vi "DiffDriveBegin.vi"(8 "error in (no error)":errorcluster) -> (0 "error out":errorcluster)   [LabVIEW 2025]
uses:
  <vilib>/Rock Robotics/WPI/ThirdParty/Phoenix-LabVIEW/Motor Controller/Controls/CTRE_Phoenix_MotorControl_NeutralMode.ctl
  <vilib>/Rock Robotics/WPI/ThirdParty/Phoenix-LabVIEW/Motor Controller/Get/CTRE_Phoenix_MotorController_GetGeneralStatus.vi
  DiffDriveGlobals.vi
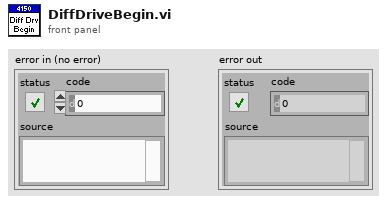
[diagram p1: front panel]
types:
  T1 = enum16{"FollowerType_PercentOutput", "FollowerType_AuxOutput1"}
  T2 = typedef "CTRE_Phoenix_MotorControl_NeutralMode.ctl" = enum8{"EEPROMSetting", "Override to Coast", "Override to Brake"}
  T3 = typedef "WPI_MotorControlDeviceRef.ctl" = cluster{"DeviceStatus":errorcluster, "Type":T4, "PWM":cluster{"PWM Channel":T5, "DeadBand":T6}, "CAN":cluster{"Device Number":u8, "SetOutput VI Ref":variant, "GetOutput VI Ref":variant, "Enable VI Ref":variant, "Disable VI Ref":variant, "Data":variant}, "Invert":bool, "DIO PWM":cluster{"PWM \"Enable\" Channel":T5, "DIOChannel":T7, "PWM Rate":dbl}}
  T4 = typedef "WPI_MotorControlType.ctl" = enum16{"PWM", "CAN", "DIO PWM"}
  T5 = typedef "FPGA_DIOPWMChannel.ctl" = enum8{"PWM 0", "PWM 1", "PWM 2", "PWM 3", "PWM 4", "PWM 5", "PWM 6", "PWM 7", "PWM 8", "PWM 9", "PWM MXP 0", "PWM MXP 1", "PWM MXP 2", "PWM MXP 3", "PWM MXP 4", "PWM MXP 5", "PWM MXP 6", "PWM MXP 7", "PWM MXP 8", "PWM MXP 9", "Invalid"}
  T6 = typedef "WPI_PWMDeadband.ctl" = cluster{"Name":string, "maxPositivePwm":i32, "minPositivePwm":i32, "centerPwm":i32, "maxNegativePwm":i32, "minNegativePwm":i32, "angularRange":u16}
  T7 = typedef "FPGA_DIOChannel.ctl" = enum8{"DIO 0", "DIO 1", "DIO 2", "DIO 3", "DIO 4", "DIO 5", "DIO 6", "DIO 7", "DIO 8", "DIO 9", "DIO MXP 0", "DIO MXP 1", "DIO MXP 2", "DIO MXP 3", "DIO MXP 4", "DIO MXP 5", "DIO MXP 6", "DIO MXP 7", "DIO MXP 8", "DIO MXP 9", "DIO MXP 10", "DIO MXP 11", "DIO MXP 12", "DIO MXP 13", "DIO MXP 14", "DIO MXP 15", "SPI Port CS1", "SPI Port CS2", "SPI Port CS3", "SPI Port MISO", "SPI Port MOSI", "Invalid"}
  T8 = typedef "ADIS16470 Device Reference.ctl" = cluster{"DevStatus":errorcluster, "Hardware Config":T9, "Calibration Complete":refnum<notifier>, "Status Reference":refnum<data-value>, "Data Reference":refnum<data-value>, "Sychronous Process VI":T12, "Cmd FIFO":refnum<k33>, "Source":T13, "Data FIFO":refnum<k33>, "Calibration Time (ms)":u32, "Data Reference":refnum<data-value>}
  T9 = typedef "ADIS16470 Hardware Configuration.ctl" = cluster{"SPI Clock Rate (Hz)":dbl, "IMU SPI Mode (3)":T10, "IMU Reset Pin":T7, "IMU SPI Bus":T11, "IMU Data Ready Pin":T7, "Stall Config":cluster{"Pow2BytesPerRead":u8, "StallTicks":u16, "CsToSclkTicks":u8}}
  T10 = typedef "WPI_SPIMode.ctl" = enum16{"Mode 0 (Clk Idle Low,Sample on Leading)", "Mode 1 (Clk Idle Low,Sample on Trailing)", "Mode 2 (Clk Idle High,Sample on Leading)", "Mode 3 (Clk Idle High,Sample on Trailing)"}
  T11 = typedef "spi_bus.ctl" = enum16{"SPI On-Board, CS0", "SPI On-Board, CS1", "SPI On-Board, CS2", "SPI On-Board, CS3", "SPI MXP", "Invalid"}
  T12 = typedef "ADIS16470 Process.ctl" = refnum<vi>
  T13 = typedef "FPGA_CounterEncoderSourceConvertionLVSourceType.ctl" = cluster{"DevStatus":errorcluster, "AnalogTriggerMode?":bool, "DigitalMode":cluster{"DIO Channel":T14}, "AnalogTriggerMode":cluster{"AnalogTriggerIndex":T15, "OutputType":T16}}
  T14 = typedef "FPGA_DIODigitalSourceChannel.ctl" = enum8{"DIO 0", "DIO 1", "DIO 2", "DIO 3", "DIO 4", "DIO 5", "DIO 6", "DIO 7", "DIO 8", "DIO 9", "DIO MXP 0", "DIO MXP 1", "DIO MXP 2", "DIO MXP 3", "DIO MXP 4", "DIO MXP 5", "DIO MXP 6", "DIO MXP 7", "DIO MXP 8", "DIO MXP 9", "DIO MXP 10", "DIO MXP 11", "DIO MXP 12", "DIO MXP 13", "DIO MXP 14", "DIO MXP 15", "SPI Port CS1", "SPI Port CS2", "SPI Port CS3", "SPI Port MISO", "SPI Port MOSI", "Disabled"}
  T15 = typedef "FPGA_AnalogTriggerIndex.ctl" = enum8{"Trig 0", "Trig 1", "Trig 2", "Trig 3", "Trig 4", "Trig 5", "Trig 6", "Trig 7", "Invalid"}
  T16 = typedef "FPGA_AnalogTriggerOutType.ctl" = enum16{"InWindow", "TriggerState", "Rising", "Falling"}
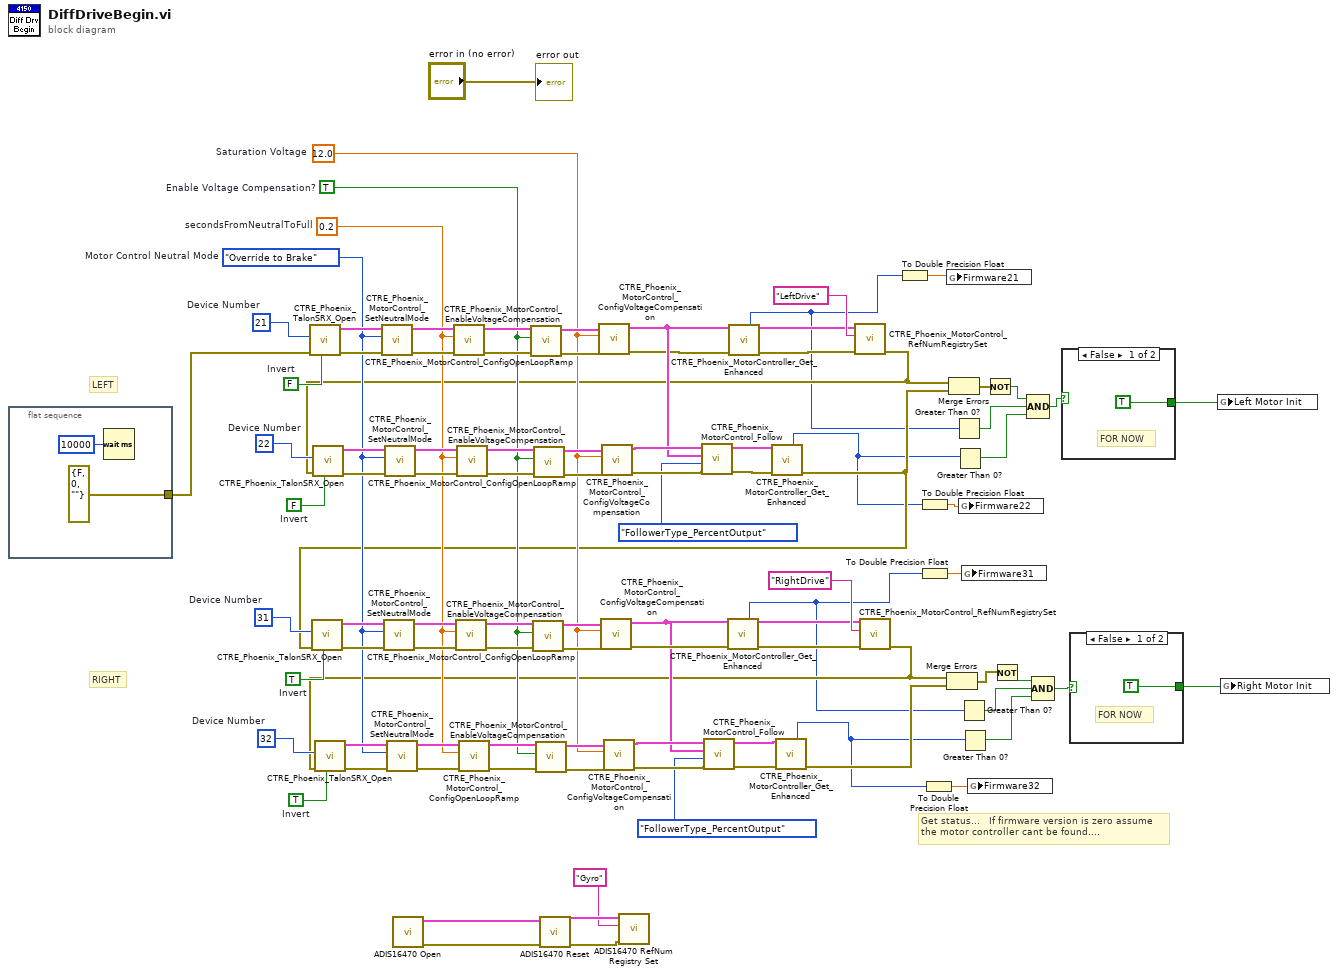
[diagram p0: block diagram]
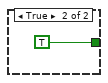
[diagram p2: hidden frame]
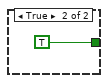
[diagram p3: hidden frame]
diagram:
  w61 = TRUE  # Invert
  w62 = u8 32  # Device Number
  w70 = TRUE  # Invert
  w71 = u8 31  # Device Number
  w84 = FALSE  # Invert
  w85 = u8 22  # Device Number
  w44 = 12.0  # Saturation Voltage
  w45 = TRUE  # Enable Voltage Compensation?
  w46 = 0.2  # secondsFromNeutralToFull
  w48 = CTRE_Phoenix_MotorControl_NeutralMode."Override to Brake"  # Motor Control Neutral Mode
  w94 = FALSE  # Invert
  w95 = u8 21  # Device Number
  # "Get status...   If firmware version is zero assume\nthe motor controller cant be found...."
  # "RIGHT"
  # "LEFT"
  n1 = flat-sequence {
    tunnel: [errorcluster {"status"=FALSE, "code"=0, "source"=""} ("error constant")] -> w14
    frame #0 {
      n2 = Wait (ms)(milliseconds to wait=u32 10000) -> ()  [unwired: 1 out]
    }
  }
  n3 = call <vilib>:"CTRE_Phoenix_TalonSRX_Open.vi"("Invert"=w94, "error in"=w14, "Device Number"=w95) -> ("error out"=w92:errorcluster, "PhoenixMotorControlDevRef"=w93:T3)  [unwired: 7 in]
  n4 = call <vilib>:"CTRE_Phoenix_MotorControl_SetNeutralMode.vi"("error in (no error)"=w92, "Motor Control Neutral Mode"=w48, "PhoenixMotorControlDevRef"=w93) -> ("error out"=w76:errorcluster, "PhoenixMotorControlDevRef"=w91:T3)  [unwired: 7 in]
  n5 = call <vilib>:"ADIS16470 Open.vi"() -> ("error out"=w5:errorcluster, "ADIS16470DevRef"=w2:T8)  [unwired: 10 in]
  n6 = call <vilib>:"CTRE_Phoenix_MotorControl_ConfigOpenLoopRamp.vi"("error in (no error)"=w76, "secondsFromNeutralToFull"=w46, "PhoenixMotorControlDevRef"=w91) -> ("error out"=w89:errorcluster, "PhoenixMotorControlDevRef"=w90:T3)  [unwired: 7 in]
  n7 = call <vilib>:"CTRE_Phoenix_MotorControl_EnableVoltageCompensation.vi"("error in (no error)"=w89, "Enable Voltage Compensation?"=w45, "PhoenixMotorControlDevRef"=w90) -> ("error out"=w87:errorcluster, "PhoenixMotorControlDevRef"=w88:T3)  [unwired: 7 in]
  n8 = call <vilib>:"ADIS16470 Reset.vi"("error in (no error)"=w5, "ADIS16470DevRef"=w2) -> ("error out"=w4:errorcluster, "ADIS16470DevRef"=w3:T8)  [unwired: 8 in]
  n9 = call <vilib>:"CTRE_Phoenix_MotorControl_ConfigVoltageCompensation.vi"("error in (no error)"=w87, "Saturation Voltage"=w44, "PhoenixMotorControlDevRef"=w88) -> ("error out"=w39:errorcluster, "PhoenixMotorControlDevRef"=w40:T3)  [unwired: 7 in]
  n10 = call <vilib>:"ADIS16470 RefNum Registry Set.vi"("error in (no error)"=w4, "refnum name"="Gyro", "ADIS16470DevRef in"=w3) -> ()  [unwired: 7 in, 2 out]
  n11 = call-poly <vilib>:"CTRE_Phoenix_MotorController_Get_Enhanced.vi"("PhoenixMotorControlDevRef"=w40, "error in"=w39) -> ("Firmware Version"=w9:i32, "PhoenixMotorControlDevRef"=w38:T3, "error out"=w37:errorcluster)  [unwired: 8 in, 3 out]
  n12 = call <vilib>:"CTRE_Phoenix_MotorControl_RefNumRegistrySet.vi"("error in (no error)"=w37, "refnum name"="LeftDrive", "PhoenixMotorControlDevRef"=w38) -> ("error out"=w17:errorcluster)  [unwired: 7 in, 1 out]
  n13 = call <vilib>:"CTRE_Phoenix_TalonSRX_Open.vi"("Invert"=w84, "error in"=w17, "Device Number"=w85) -> ("error out"=w82:errorcluster, "PhoenixMotorControlDevRef"=w83:T3)  [unwired: 7 in]
  n14 = call <vilib>:"CTRE_Phoenix_MotorControl_SetNeutralMode.vi"("error in (no error)"=w82, "Motor Control Neutral Mode"=w48, "PhoenixMotorControlDevRef"=w83) -> ("error out"=w75:errorcluster, "PhoenixMotorControlDevRef"=w81:T3)  [unwired: 7 in]
  n15 = call <vilib>:"CTRE_Phoenix_MotorControl_ConfigOpenLoopRamp.vi"("error in (no error)"=w75, "secondsFromNeutralToFull"=w46, "PhoenixMotorControlDevRef"=w81) -> ("error out"=w79:errorcluster, "PhoenixMotorControlDevRef"=w80:T3)  [unwired: 7 in]
  n16 = call <vilib>:"CTRE_Phoenix_MotorControl_EnableVoltageCompensation.vi"("error in (no error)"=w79, "Enable Voltage Compensation?"=w45, "PhoenixMotorControlDevRef"=w80) -> ("error out"=w77:errorcluster, "PhoenixMotorControlDevRef"=w78:T3)  [unwired: 7 in]
  n17 = call <vilib>:"CTRE_Phoenix_MotorControl_ConfigVoltageCompensation.vi"("error in (no error)"=w77, "Saturation Voltage"=w44, "PhoenixMotorControlDevRef"=w78) -> ("error out"=w73:errorcluster, "PhoenixMotorControlDevRef"=w74:T3)  [unwired: 7 in]
  n18 = call <vilib>:"CTRE_Phoenix_MotorControl_Follow.vi"("error in (no error)"=w73, "FollowerType"=T1."FollowerType_PercentOutput", "Master Controller to Follow"=w40, "PhoenixMotorControlDevRef"=w74) -> ("error out"=w35:errorcluster, "PhoenixMotorControlDevRef"=w36:T3)  [unwired: 6 in]
  n19 = call-poly <vilib>:"CTRE_Phoenix_MotorController_Get_Enhanced.vi"("PhoenixMotorControlDevRef"=w36, "error in"=w35) -> ("Firmware Version"=w8:i32, "error out"=w16:errorcluster)  [unwired: 8 in, 4 out]
  n20 = call <vilib>:"CTRE_Phoenix_TalonSRX_Open.vi"("Invert"=w70, "error in"=w16, "Device Number"=w71) -> ("error out"=w68:errorcluster, "PhoenixMotorControlDevRef"=w69:T3)  [unwired: 7 in]
  n21 = call <vilib>:"CTRE_Phoenix_MotorControl_SetNeutralMode.vi"("error in (no error)"=w68, "Motor Control Neutral Mode"=w48, "PhoenixMotorControlDevRef"=w69) -> ("error out"=w53:errorcluster, "PhoenixMotorControlDevRef"=w67:T3)  [unwired: 7 in]
  n22 = call <vilib>:"CTRE_Phoenix_MotorControl_ConfigOpenLoopRamp.vi"("error in (no error)"=w53, "secondsFromNeutralToFull"=w46, "PhoenixMotorControlDevRef"=w67) -> ("error out"=w65:errorcluster, "PhoenixMotorControlDevRef"=w66:T3)  [unwired: 7 in]
  n23 = call <vilib>:"CTRE_Phoenix_MotorControl_EnableVoltageCompensation.vi"("error in (no error)"=w65, "Enable Voltage Compensation?"=w45, "PhoenixMotorControlDevRef"=w66) -> ("error out"=w63:errorcluster, "PhoenixMotorControlDevRef"=w64:T3)  [unwired: 7 in]
  n24 = call <vilib>:"CTRE_Phoenix_MotorControl_ConfigVoltageCompensation.vi"("error in (no error)"=w63, "Saturation Voltage"=w44, "PhoenixMotorControlDevRef"=w64) -> ("error out"=w34:errorcluster, "PhoenixMotorControlDevRef"=w33:T3)  [unwired: 7 in]
  n25 = call-poly <vilib>:"CTRE_Phoenix_MotorController_Get_Enhanced.vi"("PhoenixMotorControlDevRef"=w33, "error in"=w34) -> ("Firmware Version"=w7:i32, "PhoenixMotorControlDevRef"=w32:T3, "error out"=w31:errorcluster)  [unwired: 8 in, 3 out]
  n26 = call <vilib>:"CTRE_Phoenix_MotorControl_RefNumRegistrySet.vi"("error in (no error)"=w31, "refnum name"="RightDrive", "PhoenixMotorControlDevRef"=w32) -> ("error out"=w15:errorcluster)  [unwired: 7 in, 1 out]
  n27 = call <vilib>:"CTRE_Phoenix_TalonSRX_Open.vi"("Invert"=w61, "error in"=w15, "Device Number"=w62) -> ("error out"=w59:errorcluster, "PhoenixMotorControlDevRef"=w60:T3)  [unwired: 7 in]
  n28 = call <vilib>:"CTRE_Phoenix_MotorControl_SetNeutralMode.vi"("error in (no error)"=w59, "Motor Control Neutral Mode"=w48, "PhoenixMotorControlDevRef"=w60) -> ("error out"=w52:errorcluster, "PhoenixMotorControlDevRef"=w58:T3)  [unwired: 7 in]
  n29 = call <vilib>:"CTRE_Phoenix_MotorControl_ConfigOpenLoopRamp.vi"("error in (no error)"=w52, "secondsFromNeutralToFull"=w46, "PhoenixMotorControlDevRef"=w58) -> ("error out"=w56:errorcluster, "PhoenixMotorControlDevRef"=w57:T3)  [unwired: 7 in]
  n30 = call <vilib>:"CTRE_Phoenix_MotorControl_EnableVoltageCompensation.vi"("error in (no error)"=w56, "Enable Voltage Compensation?"=w45, "PhoenixMotorControlDevRef"=w57) -> ("error out"=w54:errorcluster, "PhoenixMotorControlDevRef"=w55:T3)  [unwired: 7 in]
  n31 = call <vilib>:"CTRE_Phoenix_MotorControl_ConfigVoltageCompensation.vi"("error in (no error)"=w54, "Saturation Voltage"=w44, "PhoenixMotorControlDevRef"=w55) -> ("error out"=w50:errorcluster, "PhoenixMotorControlDevRef"=w51:T3)  [unwired: 7 in]
  n32 = call <vilib>:"CTRE_Phoenix_MotorControl_Follow.vi"("error in (no error)"=w50, "FollowerType"=T1."FollowerType_PercentOutput", "Master Controller to Follow"=w33, "PhoenixMotorControlDevRef"=w51) -> ("error out"=w29:errorcluster, "PhoenixMotorControlDevRef"=w30:T3)  [unwired: 6 in]
  n33 = call-poly <vilib>:"CTRE_Phoenix_MotorController_Get_Enhanced.vi"("PhoenixMotorControlDevRef"=w30, "error in"=w29) -> ("Firmware Version"=w6:i32, "error out"=w28:errorcluster)  [unwired: 8 in, 4 out]
  n34 = To Double Precision Float(number=w9) -> (double precision float=w13:dbl)
  n35 = To Double Precision Float(number=w8) -> (double precision float=w12:dbl)
  n36 = To Double Precision Float(number=w7) -> (double precision float=w11:dbl)
  n37 = To Double Precision Float(number=w6) -> (double precision float=w10:dbl)
  n38 = global write "DiffDriveGlobals.vi" "Firmware21"(w13) -> ()
  n39 = Merge Errors(w15, w28) -> (w19:errorcluster)
  n40 = Merge Errors(w17, w16) -> (w20:errorcluster)
  n41 = Greater Than 0?(x=w9) -> (x > 0?=w26:bool)
  n42 = Greater Than 0?(x=w8) -> (x > 0?=w25:bool)
  n43 = global write "DiffDriveGlobals.vi" "Firmware22"(w12) -> ()
  n44 = Greater Than 0?(x=w7) -> (x > 0?=w22:bool)
  n45 = Greater Than 0?(x=w6) -> (x > 0?=w24:bool)
  n46 = global write "DiffDriveGlobals.vi" "Firmware31"(w11) -> ()
  n47 = global write "DiffDriveGlobals.vi" "Firmware32"(w10) -> ()
  n48 = Not(x=w20) -> (.not. x?=w21:bool)
  n49 = Not(x=w19) -> (.not. x?=w18:bool)
  n50 = Compound Arithmetic op=AND(w21, w26, w25) -> (w27:bool)
  n51 = Compound Arithmetic op=AND(w18, w22, w24) -> (w23:bool)
  n52 = case shown="False" w27 {
    tunnel: [TRUE TRUE] -> w42
    frame False {
      # "FOR NOW"
    }
    frame True {
    }
  }
  n53 = case shown="False" w23 {
    tunnel: [TRUE TRUE] -> w41
    frame False {
      # "FOR NOW"
    }
    frame True {
    }
  }
  n54 = global write "DiffDriveGlobals.vi" "Left Motor Init"(w42) -> ()
  n55 = global write "DiffDriveGlobals.vi" "Right Motor Init"(w41) -> ()
  "error out" <- "error in (no error)"
